vi "Ricalcolo gradezze n.vi"(9 "Densità per ricalcolo P2":dbl, 10 "rpm nom":dbl, 11 "MISURE NM in":T1) -> (3 "MISURE NM out":T1)   [LabVIEW 2019]
uses:
  TypeDef/MISURE NM.ctl
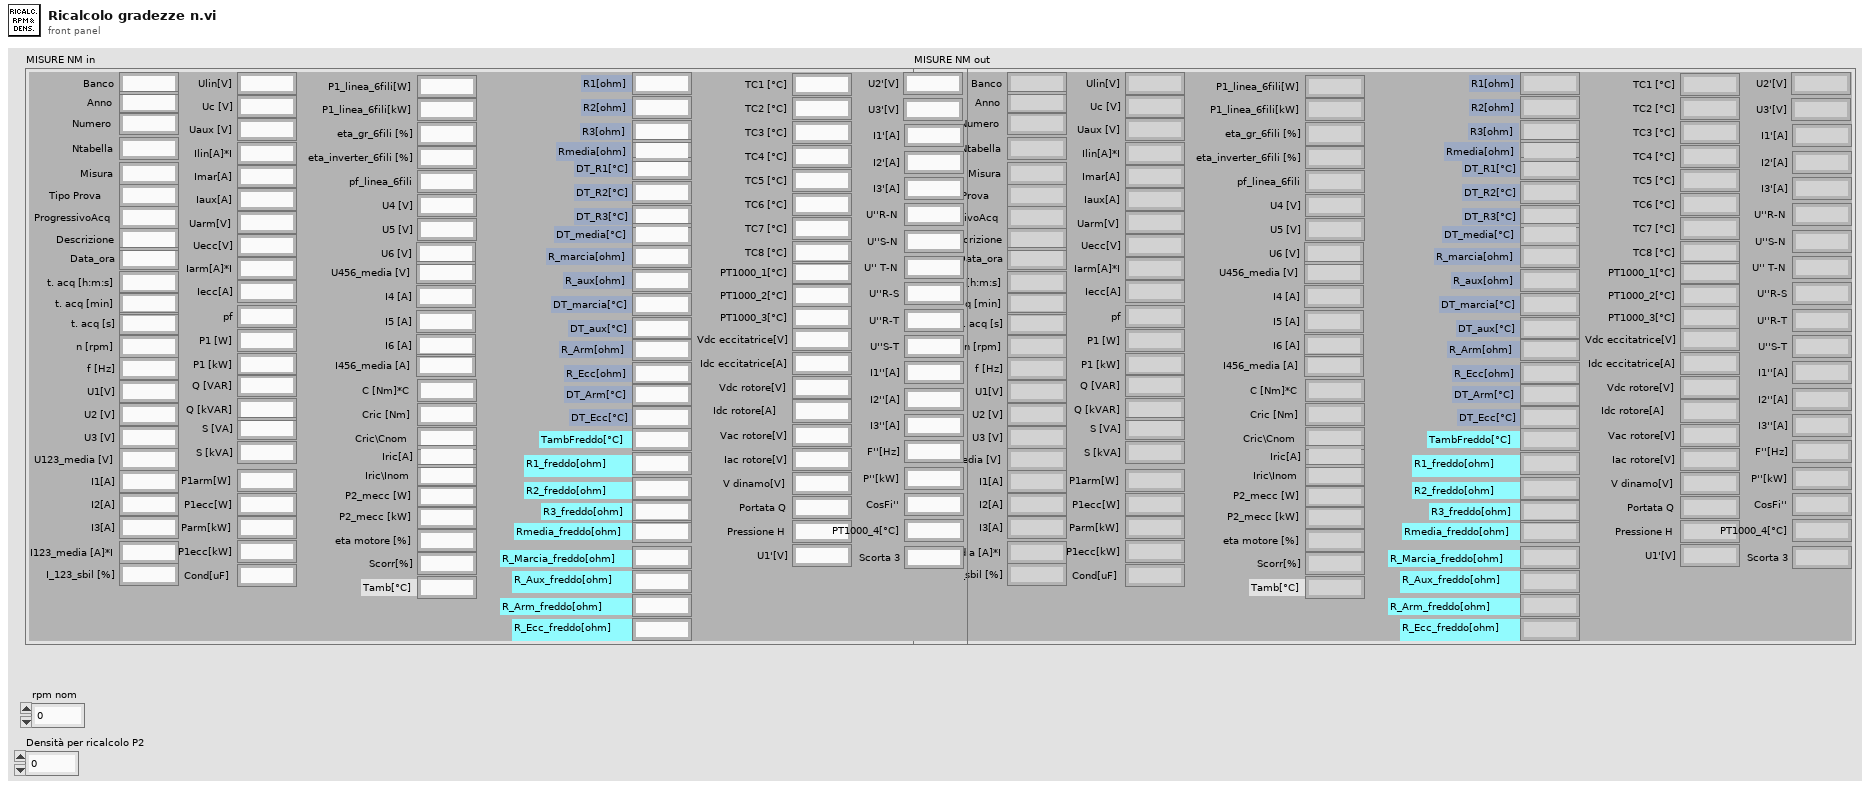
[diagram p1: front panel]
types:
  T1 = typedef "MISURE NM.ctl" = cluster{"Banco":string, "Anno":string, "Numero":string, "Ntabella":string, "Misura":string, "Tipo Prova":string, "ProgressivoAcq":string, "Descrizione":string, "Data_ora":string, "t. acq [h:m:s]":string, "t. acq [min]":string, "t. acq [s]":string, "n [rpm]":string, "f [Hz]":string, "U1[V]":string, "U2 [V]":string, "U3 [V]":string, "U123_media [V]":string, "I1[A]":string, "I2[A]":string, "I3[A]":string, "I123_media [A]*I":string, "I_123_sbil [%]":string, "Ulin[V]":string, "Uc [V]":string, "Uaux [V]":string, "Ilin[A]*I":string, "Imar[A]":string, "Iaux[A]":string, "Uarm[V]":string, "Uecc[V]":string, "Iarm[A]*I":string, "Iecc[A]":string, "pf":string, "P1 [W]":string, "P1 [kW]":string, "Q [VAR]":string, "Q [kVAR]":string, "S [VA]":string, "S [kVA]":string, "P1arm[W]":string, "P1ecc[W]":string, "Parm[kW]":string, "P1ecc[kW]":string, "Cond[uF]":string, "P1_linea_6fili[W]":string, "P1_linea_6fili[kW]":string, "eta_gr_6fili [%]":string, "eta_inverter_6fili [%]":string, "pf_linea_6fili":string, "U4 [V]":string, "U5 [V]":string, "U6 [V]":string, "U456_media [V]":string, "I4 [A]":string, "I5 [A]":string, "I6 [A]":string, "I456_media [A]":string, "C [Nm]*C":string, "Cric [Nm]":string, "Cric\\Cnom":string, "Iric[A]":string, "Iric\\Inom":string, "P2_mecc [W]":string, "P2_mecc [kW]":string, "eta motore [%]":string, "Scorr[%]":string, "Tamb[°C]":string, "R1[ohm]":string, "R2[ohm]":string, "R3[ohm]":string, "Rmedia[ohm]":string, "DT_R1[°C]":string, "DT_R2[°C]":string, "DT_R3[°C]":string, "DT_media[°C]":string, "R_marcia[ohm]":string, "R_aux[ohm]":string, "DT_marcia[°C]":string, "DT_aux[°C]":string, "R_Arm[ohm]":string, "R_Ecc[ohm]":string, "DT_Arm[°C]":string, "DT_Ecc[°C]":string, "TambFreddo[°C]":string, "R1_freddo[ohm]":string, "R2_freddo[ohm]":string, "R3_freddo[ohm]":string, "Rmedia_freddo[ohm]":string, "R_Marcia_freddo[ohm]":string, "R_Aux_freddo[ohm]":string, "R_Arm_freddo[ohm]":string, "R_Ecc_freddo[ohm]":string, "TC1 [°C]":string, "TC2 [°C]":string, "TC3 [°C]":string, "TC4 [°C]":string, "TC5 [°C]":string, "TC6 [°C]":string, "TC7 [°C]":string, "TC8 [°C]":string, "PT1000_1[°C]":string, "PT1000_2[°C]":string, "PT1000_3[°C]":string, "Vdc eccitatrice[V]":string, "Idc eccitatrice[A]":string, "Vdc rotore[V]":string, "Idc rotore[A]":string, "Vac rotore[V]":string, "Iac rotore[V]":string, "V dinamo[V]":string, "Portata Q":string, "Pressione H":string, "U1'[V]":string, "U2'[V]":string, "U3'[V]":string, "I1'[A]":string, "I2'[A]":string, "I3'[A]":string, "U''R-N":string, "U''S-N":string, "U'' T-N":string, "U''R-S":string, "U''R-T":string, "U''S-T":string, "I1''[A]":string, "I2''[A]":string, "I3''[A]":string, "F''[Hz]":string, "P''[kW]":string, "CosFi''":string, "PT1000_4[°C]":string, "Scorta 3":string}
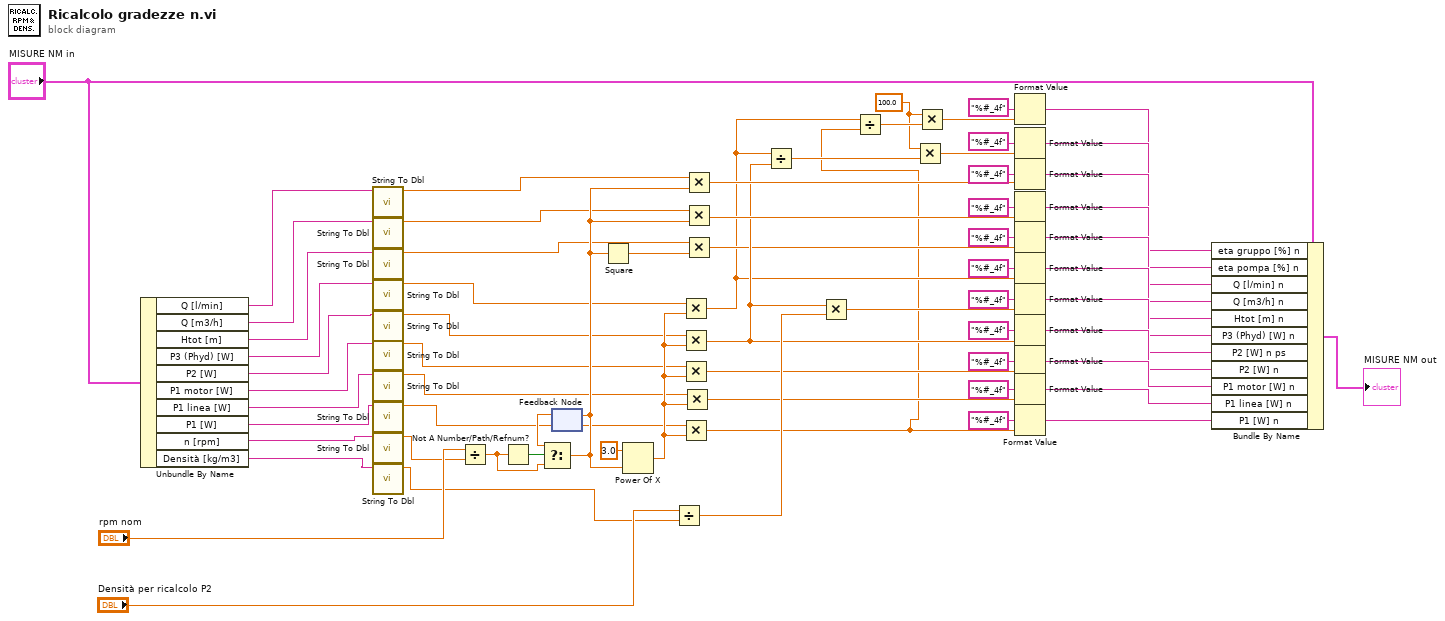
[diagram p0: block diagram]
diagram:
  w22 = 100.0 ("x")
  n1 = Unbundle By Name("MISURE NM in") -> ("Q [l/min]"=w20:string, "Q [m3/h]"=w18:string, "Htot [m]"=w1:string, "P3 (Phyd) [W]"=w15:string, "P2 [W]"=w13:string, "P1 motor [W]"=w11:string, "P1 linea [W]"=w9:string, "P1 [W]"=w7:string, "n [rpm]"=w5:string, "Densità [kg/m3]"=w3:string)
  n2 = call "String To Dbl.vi"("String"=w20) -> ("Numeric"=w19:dbl)  [unwired: 10 in]
  n3 = call "String To Dbl.vi"("String"=w18) -> ("Numeric"=w17:dbl)  [unwired: 10 in]
  n4 = call "String To Dbl.vi"("String"=w1) -> ("Numeric"=w16:dbl)  [unwired: 10 in]
  n5 = call "String To Dbl.vi"("String"=w15) -> ("Numeric"=w14:dbl)  [unwired: 10 in]
  n6 = call "String To Dbl.vi"("String"=w13) -> ("Numeric"=w12:dbl)  [unwired: 10 in]
  n7 = call "String To Dbl.vi"("String"=w11) -> ("Numeric"=w10:dbl)  [unwired: 10 in]
  n8 = call "String To Dbl.vi"("String"=w9) -> ("Numeric"=w8:dbl)  [unwired: 10 in]
  n9 = call "String To Dbl.vi"("String"=w7) -> ("Numeric"=w6:dbl)  [unwired: 10 in]
  n10 = call "String To Dbl.vi"("String"=w5) -> ("Numeric"=w4:dbl)  [unwired: 10 in]
  n11 = call "String To Dbl.vi"("String"=w3) -> ("Numeric"=w2:dbl)  [unwired: 10 in]
  n12 = Divide(x="rpm nom", y=w4) -> (x/y=w49:dbl)
  n13 = Not A Number/Path/Refnum?(number/path/refnum=w49) -> (NaN/Path/Refnum?=w51:bool)
  n14 = feedback #1() -> (w50:dbl)  [unwired: 1 in]
  n15 = Select(t=w50, s=w51, f=w49) -> (s? t:f=w39:dbl)
  n16 = feedback-in #1(w39) -> ()
  n17 = Square(x=w39) -> (x^2=w44:dbl)
  n18 = Power Of X(1:w39, 2:3.0 ("x")) -> (0:w48:dbl)
  n19 = Divide(x="Densità per ricalcolo P2", y=w2) -> (x/y=w58:dbl)
  n20 = Multiply(x=w14, y=w48) -> (x*y=w26:dbl)
  n21 = Multiply(x=w12, y=w48) -> (x*y=w35:dbl)
  n22 = Multiply(x=w10, y=w48) -> (x*y=w30:dbl)
  n23 = Multiply(x=w6, y=w48) -> (x*y=w21:dbl)
  n24 = Multiply(x=w8, y=w48) -> (x*y=w31:dbl)
  n25 = Multiply(x=w19, y=w39) -> (x*y=w37:dbl)
  n26 = Multiply(x=w17, y=w39) -> (x*y=w41:dbl)
  n27 = Multiply(x=w16, y=w44) -> (x*y=w32:dbl)
  n28 = Divide(x=w26, y=w35) -> (x/y=w24:dbl)
  n29 = Multiply(x=w35, y=w58) -> (x*y=w55:dbl)
  n30 = Divide(x=w26, y=w21) -> (x/y=w28:dbl)
  n31 = Multiply(x=w22, y=w24) -> (x*y=w23:dbl)
  n32 = Multiply(x=w22, y=w28) -> (x*y=w25:dbl)
  n33 = Format Value(format string="%#_4f", value (0)=w25) -> (output string=w27:string)  [unwired: 1 in]
  n34 = Format Value(format string="%#_4f", value (0)=w23) -> (output string=w33:string)  [unwired: 1 in]
  n35 = Format Value(format string="%#_4f", value (0)=w37) -> (output string=w36:string)  [unwired: 1 in]
  n36 = Format Value(format string="%#_4f", value (0)=w41) -> (output string=w40:string)  [unwired: 1 in]
  n37 = Format Value(format string="%#_4f", value (0)=w32) -> (output string=w43:string)  [unwired: 1 in]
  n38 = Format Value(format string="%#_4f", value (0)=w26) -> (output string=w46:string)  [unwired: 1 in]
  n39 = Format Value(format string="%#_4f", value (0)=w55) -> (output string=w54:string)  [unwired: 1 in]
  n40 = Format Value(format string="%#_4f", value (0)=w35) -> (output string=w59:string)  [unwired: 1 in]
  n41 = Format Value(format string="%#_4f", value (0)=w30) -> (output string=w61:string)  [unwired: 1 in]
  n42 = Format Value(format string="%#_4f", value (0)=w31) -> (output string=w63:string)  [unwired: 1 in]
  n43 = Format Value(format string="%#_4f", value (0)=w21) -> (output string=w67:string)  [unwired: 1 in]
  n44 = Bundle By Name(cluster="MISURE NM in", "eta gruppo [%] n"=w27, "eta pompa [%] n"=w33, "Q [l/min] n"=w36, "Q [m3/h] n"=w40, "Htot [m] n"=w43, "P3 (Phyd) [W] n"=w46, "P2 [W] n ps"=w54, "P2 [W] n"=w59, "P1 motor [W] n"=w61, "P1 linea [W] n"=w63, "P1 [W] n"=w67) -> (→"MISURE NM out":T1)
